vi "ArmGoalEndEffectorPosition.vi"(1 "Goal Wrist Angle (deg)":dbl, 2 "Goal Elbow Angle (deg)":dbl, 3 "Goal Shoulder Angle (deg)":dbl) -> (0 "Translation Vector (in)":dbl[](array[numeric]))   [LabVIEW 2020]
doc: "Calculates the goal end effector position based on the goal arm joint angles."
uses:
  <vilib>/robotics/Kinematics/NI_Kinematics.lvlib
  GlobalArm.vi
  <vilib>/robotics/Kinematics/Robot/Forward Kinematics (Point).vi
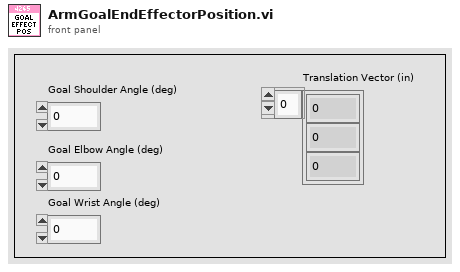
[diagram p1: front panel]
types:
  T1 = typedef "NI_Matrix.lvlib/RealMatrix.ctl" = dbl[][]
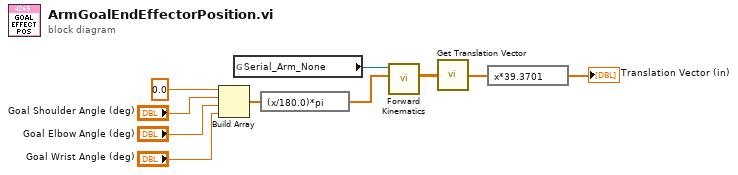
[diagram p0: block diagram]
diagram:
  n1 = Build Array(0.0 ("element"), "Goal Shoulder Angle (deg)", "Goal Elbow Angle (deg)", "Goal Wrist Angle (deg)") -> (w8:dbl[])
  n2 = global read "GlobalArm.vi" "Serial_Arm_None"() -> (w3:refnum<class "NI_Robotics_Serial Robot Arm.lvclass">)
  n3 = expression code="(x/180.0)*pi" ("degrees to radians")(w8) -> (w9:dbl[])
  n4 = call-poly <vilib>:"Forward Kinematics.vi"("joint positions"=w9, "serial arm in"=w3) -> ("end effector transform"=w10:T1)  [unwired: 7 in, 2 out]
  n5 = call <vilib>:"Get Translation Vector.vi"("transform"=w10) -> ("translation vector"=w2:dbl[])
  n6 = expression code="x*39.3701" ("degrees to radians")(w2) -> (→"Translation Vector (in)":dbl[])
